vi "RPC Close App Reference.vi"(8 "error in (no error)":errorcluster, 11 "app reference":refnum<vi>) -> (0 "error out":errorcluster)   [LabVIEW 2011]
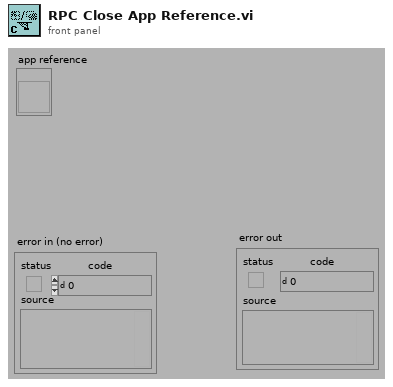
[diagram p1: front panel]
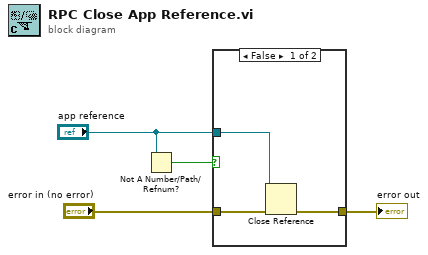
[diagram p0: block diagram]
diagram:
  n1 = Not A Number/Path/Refnum?(number/path/refnum="app reference") -> (NaN/Path/Refnum?=w2:bool)
  n2 = case shown="False" w2 {
    tunnel: "error in (no error)" -> [w7 w8]
    tunnel: [w6 w8] -> w3
    tunnel: "app reference" -> [w5 _]
    frame False {
      n3 = Close Reference(reference=w5, error in (no error)=w7) -> (error out=w6:errorcluster)
    }
    frame True {
    }
  }
  "error out" <- w3
